vi "PH_Sound.PC Laserfreigabe ein.vi"(0 "i ref in":refnum<vi>, 5 "error IO":errorcluster) -> (14 "i ref out":refnum<vi>, 19 "error out":errorcluster)   [LabVIEW 2014, in "PH_Sound.lvlib"]
doc: "This is a certain proc case."
uses:
  PH_Sound.lvlib
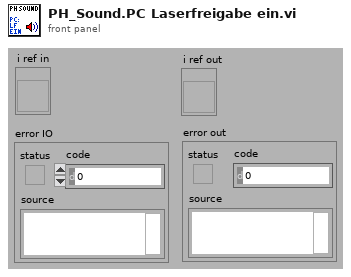
[diagram p1: front panel]
types:
  T1 = typedef "PH_Sound.lvlib/PH_Sound.i attribute.ctl" = cluster{"GUI Refs":cluster{"Exit":refnum<vi>, "Laserfreigabe":refnum<vi>, "PreAmp-Freigabe":refnum<vi>, "Countdown Running":refnum<vi>, "Emergency Off":refnum<vi>, "Device Error":refnum<vi>}, "Testalarm on":bool, "State":cluster{"Laser Class 4":bool, "PreAmp Running":bool, "Countdown Running":bool, "Emergency Off":bool}, "Starting Time":timestamp}
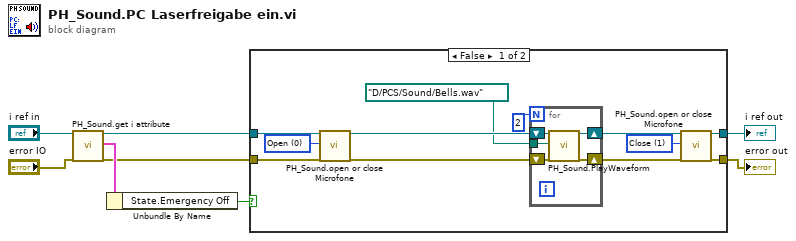
[diagram p0: block diagram]
diagram:
  n1 = call "PH_Sound.get i attribute.vi"("i ref in"="i ref in", "error in (no error)"="error IO") -> ("i ref out"=w4:refnum<vi>, "i attribute"=w5:T1, "error out"=w2:errorcluster)  [unwired: 15 in]
  n2 = Unbundle By Name(w5) -> ("State.Emergency Off"=w6:bool)
  n3 = case shown="False" w6 {
    tunnel: [w12 w27] -> w8
    tunnel: [w14 w26] -> w7
    tunnel: w2 -> [w18 w26]
    tunnel: w4 -> [w20 w27]
    frame False {
      w11 = u16 1 items=["Open", "Close"] ("Action")
      w16 = u16 0 items=["Open", "Close"] ("Action")
      n4 = call "PH_Sound.open or close Microfone.vi"("i ref in"=w20, "Action"=w16, "error in (no error)"=w18) -> ("i ref out"=w19:refnum<vi>, "error out"=w17:errorcluster)  [unwired: 15 in]
      n5 = for {
        N: 2 -> [_]
        tunnel: path "D:/PCS/Sound/Bells.wav" ("path") -> [w21]
        shift-right: [w22] -> w13
        shift-left: w19 -> [w23]
        shift-right: [w24] -> w15
        shift-left: w17 -> [w25]
        n6 = call "PH_Sound.PlayWaveform.vi"("i ref in"=w23, "path"=w21, "error in (no error)"=w25) -> ("i ref out"=w22:refnum<vi>, "error out"=w24:errorcluster)  [unwired: 15 in]
      }
      n7 = call "PH_Sound.open or close Microfone.vi"("i ref in"=w13, "Action"=w11, "error in (no error)"=w15) -> ("i ref out"=w12:refnum<vi>, "error out"=w14:errorcluster)  [unwired: 15 in]
    }
    frame True {
    }
  }
  "i ref out" <- w8
  "error out" <- w7
